vi "Remove-action-from-sequence.vi"(5 "Sequence index in":i32, 7 "Motor index":i32, 8 "error in (no error)":errorcluster, 11 "Available motors in":refnum<class "Motor-assembly.lvclass">) -> (0 "error out":errorcluster, 2 "Action":refnum<class "Action.lvclass">, 3 "Available motors out":refnum<class "Motor-assembly.lvclass">, 4 "Sequence index":i32)   [LabVIEW 2013, in "PowderDeposition.lvlib" / "Motor-assembly.lvclass"]
uses:
  Motor-assembly.lvclass
  Action/Action.lvclass
  Motor-assembly.lvclass/Motor-assembly.ctl
  Motor/Motor.lvclass
  Sequence/Action-sequence.lvclass
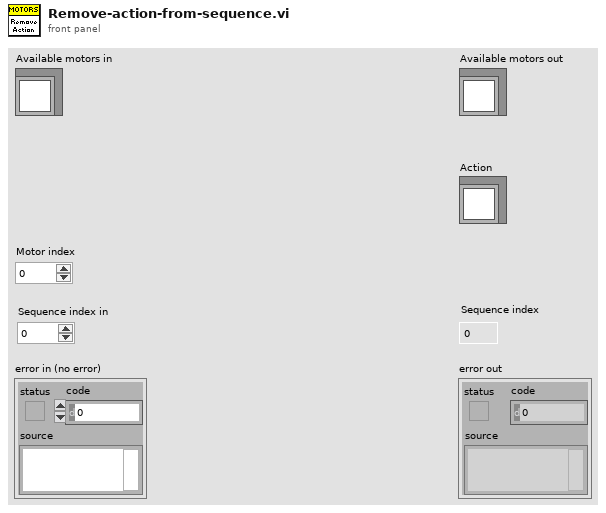
[diagram p1: front panel]
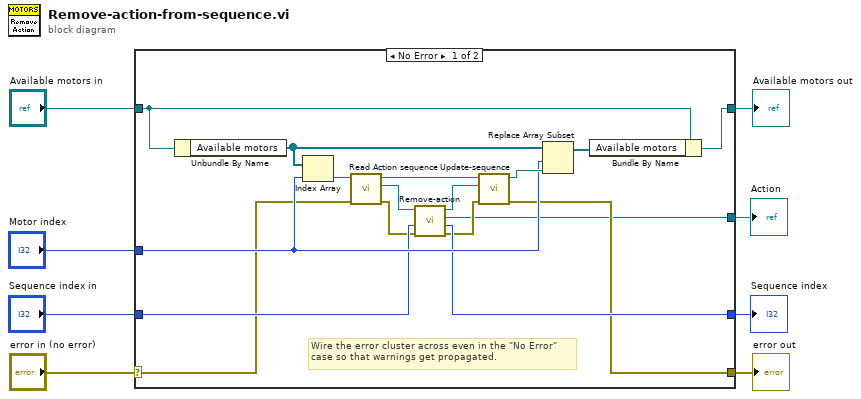
[diagram p0: block diagram]
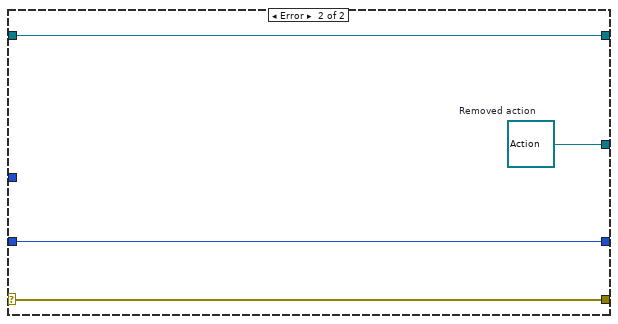
[diagram p2: hidden frame]
diagram:
  n1 = case shown="No Error" "error in (no error)" {
    selector: "error in (no error)" -> [w11 w29]
    tunnel: [w10 w29] -> w7
    tunnel: [w18 w28] -> w5
    tunnel: "Available motors in" -> [w19 w28]
    tunnel: "Motor index" -> [w17 _]
    tunnel: "Sequence index in" -> [w15 w27]
    tunnel: [w14 w27] -> w2
    tunnel: [w9 w26] -> w1
    frame No Error {
      # "Wire the error cluster across even in the \"No Error\"\ncase so that warnings get propagated."
      n2 = Unbundle By Name(w19) -> ("Available motors"=w16:refnum<class "Motor.lvclass">[])
      n3 = Index Array(array=w16, index=w17) -> (element=w21:refnum<class "Motor.lvclass">)
      n4 = call-dynamic "Read Action sequence.vi"("error in (no error)"=w11, "Motor in"=w21) -> ("error out"=w13:errorcluster, "Sequence.lvclass"=w22:refnum<class "Action-sequence.lvclass">, "Motor out"=w24:refnum<class "Motor.lvclass">)  [unwired: 7 in]
      n5 = call "Remove-action.vi"("error in (no error)"=w13, "Position in"=w15, "Sequence in"=w22) -> ("error out"=w12:errorcluster, "Position"=w14:i32, "Removed action"=w9:refnum<class "Action.lvclass">, "Sequence out"=w23:refnum<class "Action-sequence.lvclass">)  [unwired: 5 in]
      n6 = call-dynamic "Update-sequence.vi"("error in (no error)"=w12, "Sequence"=w23, "Motor in"=w24) -> ("error out"=w10:errorcluster, "Motor out"=w25:refnum<class "Motor.lvclass">)  [unwired: 7 in]
      n7 = Replace Array Subset(array=w16, new element=w25, index=w17) -> (w20:refnum<class "Motor.lvclass">[])
      n8 = Bundle By Name(cluster=w19, "Available motors"=w20) -> (w18:refnum<class "Motor-assembly.lvclass">)
    }
    frame Error {
      w26 = refnum<class "Action.lvclass"> refnum  # Removed action
    }
  }
  "error out" <- w7
  "Available motors out" <- w5
  "Action" <- w1
  "Sequence index" <- w2
